vi "sub1choice.vi"(8 "error in":errorcluster, 10 "Detector Start Pin":u8, 11 "Arduino Resource":T1={"VISA resource"="", "Board Type"=enum."Uno", "Connection Type"=enum."USB / Serial", "Bytes Per Packet (15)"=15}) -> (0 "error out":errorcluster, 2 "Numeric":dbl, 3 "Arduino Resource 2":T1={"VISA resource"="", "Board Type"=enum."Uno", "Connection Type"=enum."USB / Serial", "Bytes Per Packet (15)"=15})   [LabVIEW 2016]
uses:
  <vilib>/LabVIEW Interface for Arduino/Type Defs/Arduino Resource.ctl
  <vilib>/LabVIEW Interface for Arduino/Type Defs/Board Type.ctl
  <vilib>/LabVIEW Interface for Arduino/LabVIEW Interface for Arduino.lvlib
panel:
  out "Boolean 3":bool
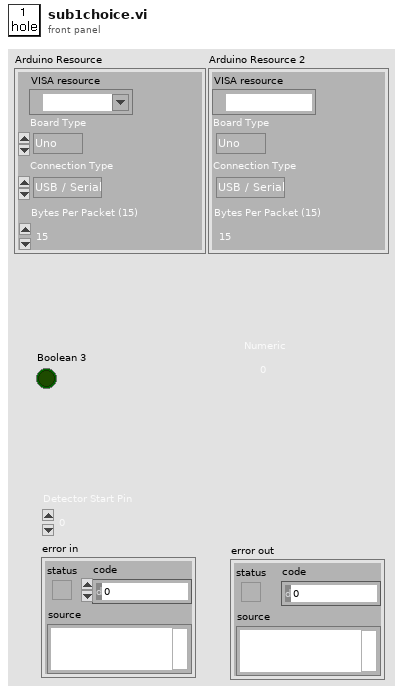
[diagram p1: front panel]
types:
  T1 = typedef "LabVIEW Interface for Arduino.lvlib/Arduino Resource.ctl" = cluster{"VISA resource":refnum<visa-resource-name>, "Board Type":T2, "Connection Type":enum8{"USB / Serial"}, "Bytes Per Packet (15)":u8}
  T2 = typedef "LabVIEW Interface for Arduino.lvlib/Board Type.ctl" = enum16{"Uno", "Dimuelanove w/Atmega 328", "Mega 2560"}
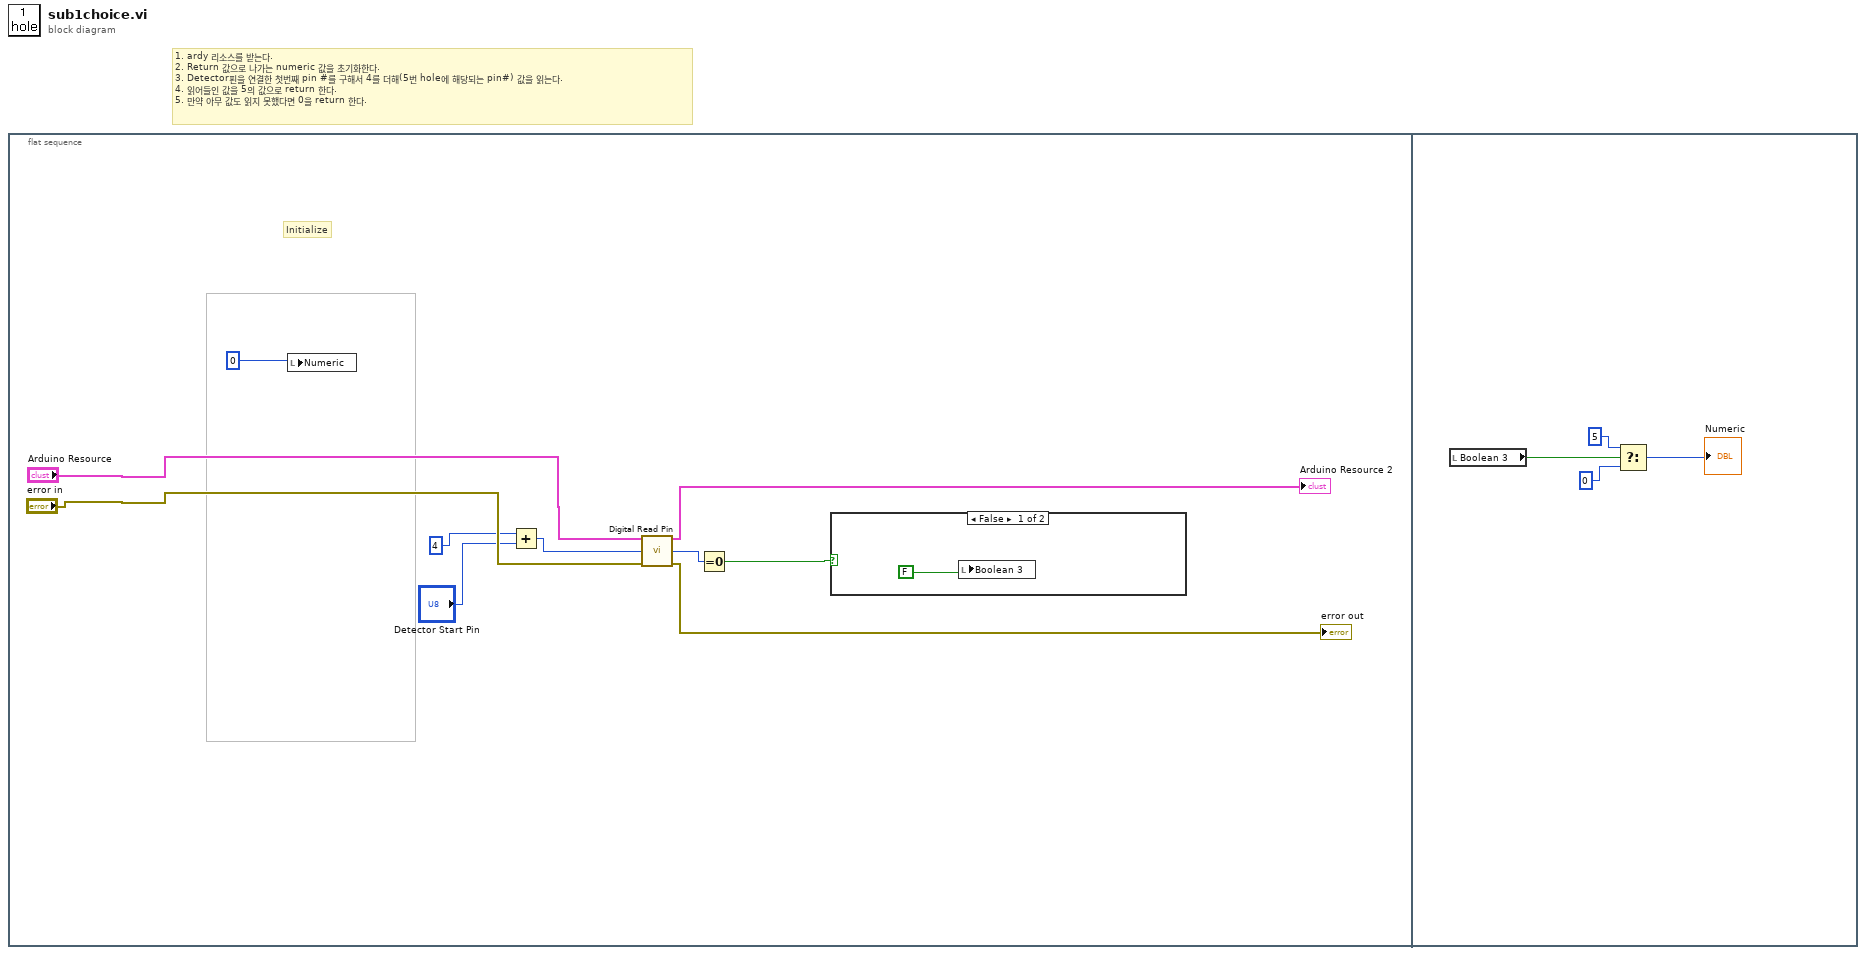
[diagram p0: block diagram]
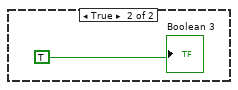
[diagram p2: hidden frame]
diagram:
  # "1. ardy 리소스를 받는다. \n2. Return 값으로 나가는 numeric 값을 초기화한다.\n3. Detector핀을 연결한 첫번째 pin #를 구해서 4를 더해(5번 hole에 해당되는 pin#) 값을 읽는다.\n4. 읽어들인 값을 5의 값으로 return 한다. \n5. 만약 아무 값도 읽지 못했다면 0을 return 한다."
  n1 = flat-sequence {
    frame #0 {
      # "Initialize"
      n2 = local write "Numeric"(0) -> ()
      n3 = Add(x=4, y="Detector Start Pin") -> (x+y=w5:i32)
      n4 = call <vilib>:"Digital Read Pin.vi"("Arduino Resource"="Arduino Resource", "Digital I/O Pin (0)"=w5, "error in"="error in") -> ("Arduino Resource"=→"Arduino Resource 2":T1, "Value"=w6:u8, "error out"=→"error out":errorcluster)  [unwired: 10 in]
      n5 = Equal To 0?(x=w6) -> (x = 0?=w7:bool)
      n6 = case shown="False" w7 {
        frame False {
          n7 = local write "Boolean 3"(FALSE) -> ()
        }
        frame True {
          "Boolean 3" <- TRUE
        }
      }
    }
    frame #1 {
      n8 = local read "Boolean 3"() -> (w16:bool)
      n9 = Select(t=5, s=w16, f=0) -> (s? t:f=→"Numeric":i32)
    }
  }
